vi "DriveFwd.vi"() -> ()   [LabVIEW 2017]
panel:
  out "drive output":dbl
  in  "Drive":dbl
  in  "SLOW?":bool
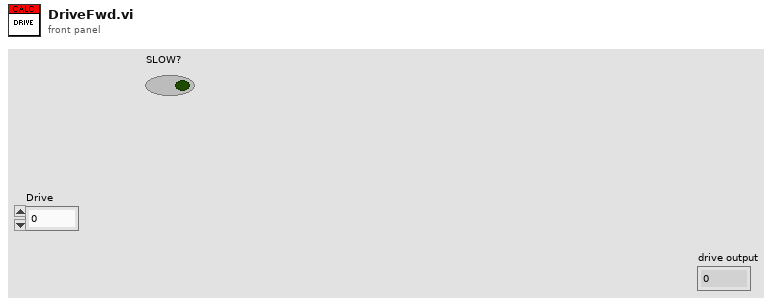
[diagram p1: front panel]
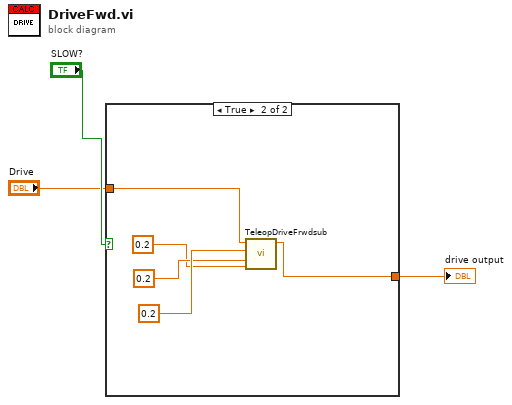
[diagram p0: block diagram]
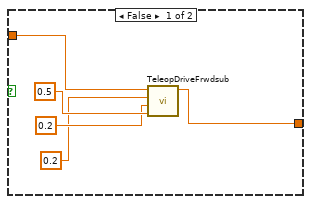
[diagram p2: hidden frame]
diagram:
  n1 = case shown="True" "SLOW?" {
    tunnel: "Drive" -> [w5 w13]
    tunnel: [w4 w12] -> w1
    frame False {
      n2 = call "TeleopDriveFrwdsub.vi"("SCALE"=0.5 ("a value"), "B VALUE"=0.2 ("b value"), "Deadband X value"=0.2 ("dead band val"), "Drive"=w5) -> ("Drive Output"=w4:dbl)  [unwired: 7 in]
    }
    frame True {
      n3 = call "TeleopDriveFrwdsub.vi"("SCALE"=0.2 ("a value"), "B VALUE"=0.2 ("b value"), "Deadband X value"=0.2 ("dead band val"), "Drive"=w13) -> ("Drive Output"=w12:dbl)  [unwired: 7 in]
    }
  }
  "drive output" <- w1
